vi "JTAG Program.vi"(7 "File format":i32(ring)=1 items=["TI "=1, "Motorola"=2, "Intel"=3], 8 "error in (no error)":errorcluster, 9 "MD5 message-digest":string, 10 "Function":T1(ring), 11 "File Path":path=path "C:/ATS Development/Code/Drivers/JTAG/JTAG Driver/Firmware/Test_Firmware_V1.txt") -> (0 "error out":errorcluster, 1 "MD5 message-digest 2":string, 3 "Status":bool)   [LabVIEW 2010]
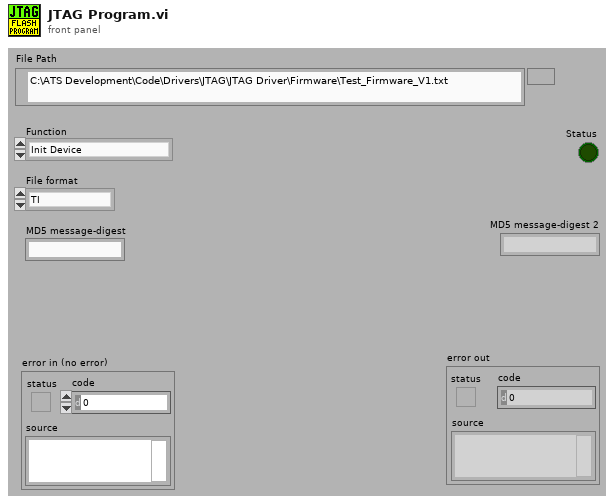
[diagram p1: front panel]
types:
  T1 = enum16{"Init Device", "Auto-Program from File", "Load New Code File", "Close Device", "Blank Check Device", "Erase Device Flash", "Program File to Flash", "Verify Flash vs File", "Read Flash to File", "Checksum of File", "Compare Checksums"}
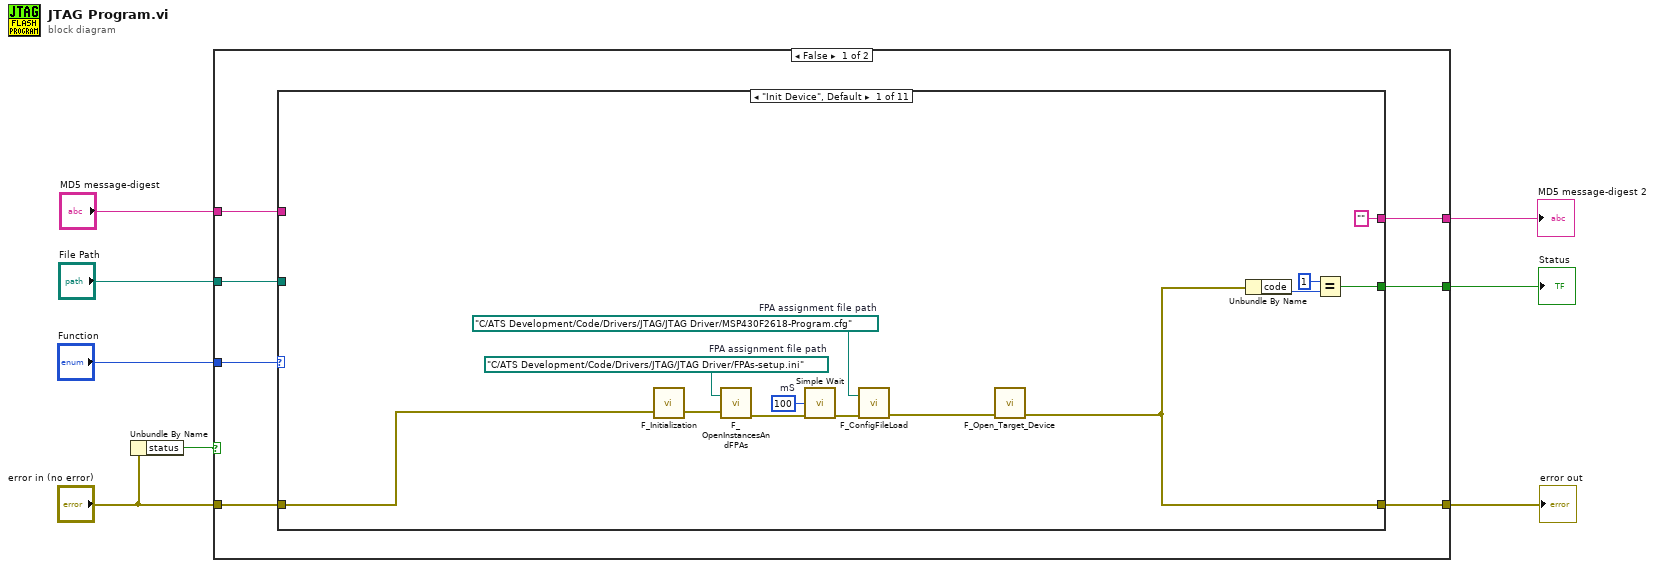
[diagram p0: block diagram]
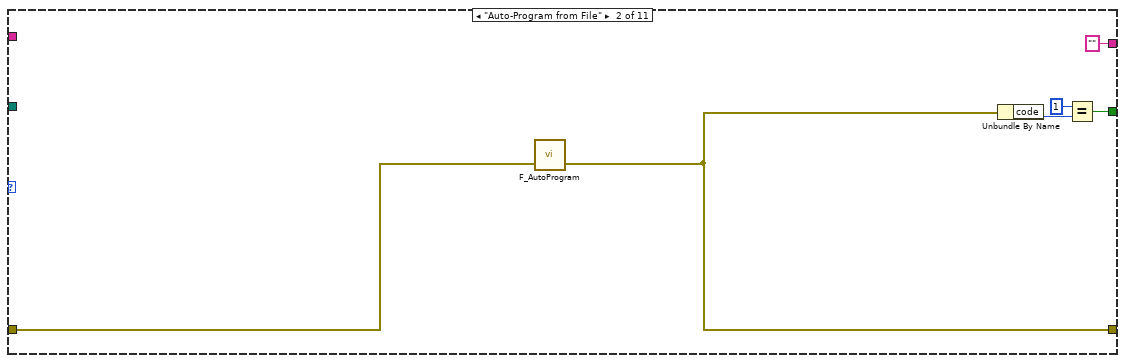
[diagram p2: hidden frame]
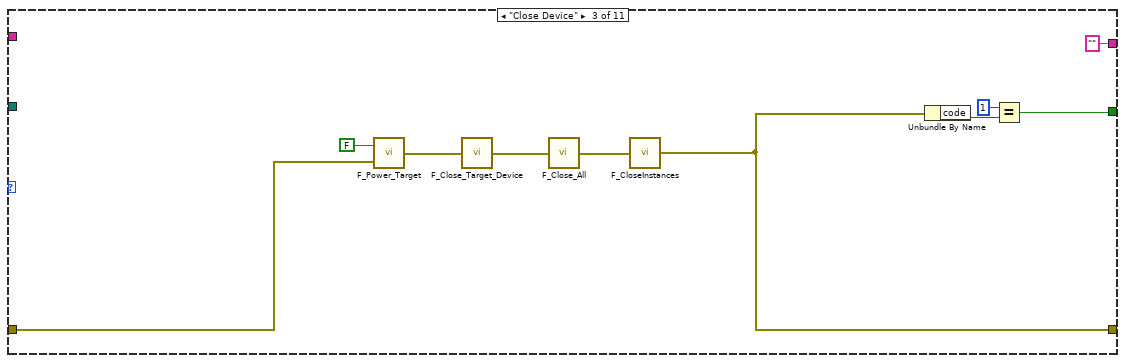
[diagram p3: hidden frame]
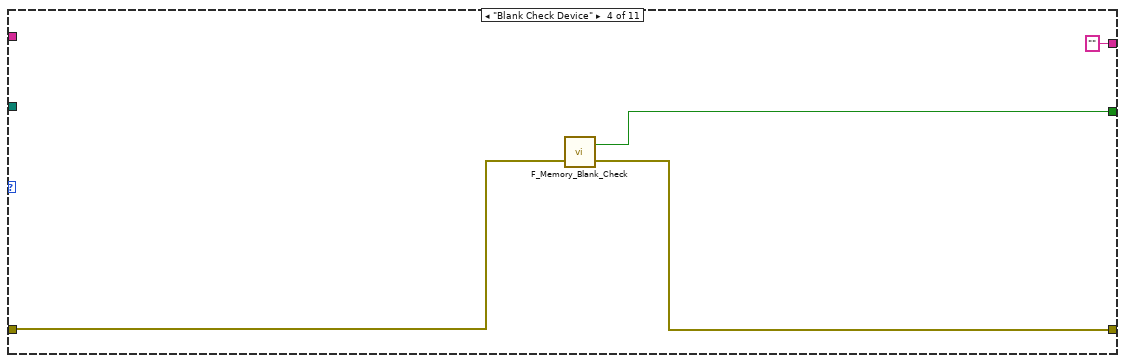
[diagram p4: hidden frame]
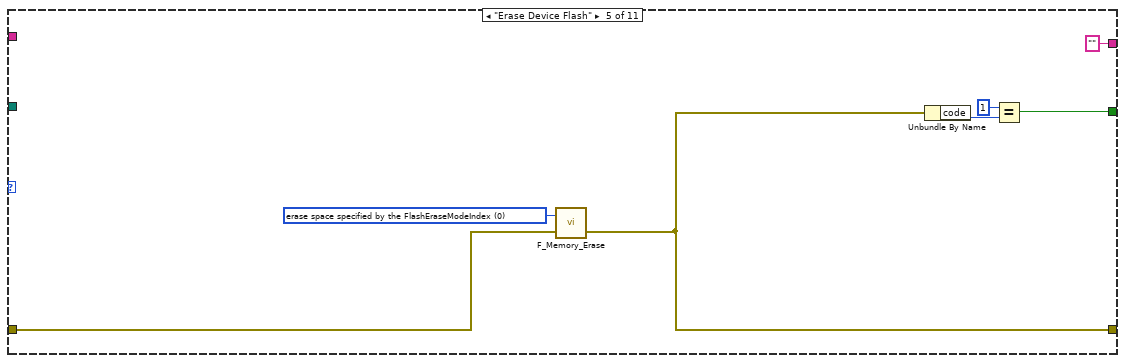
[diagram p5: hidden frame]
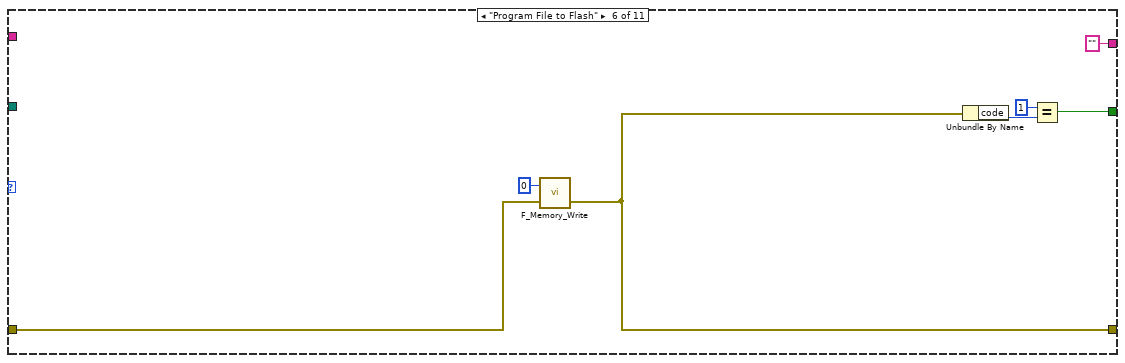
[diagram p6: hidden frame]
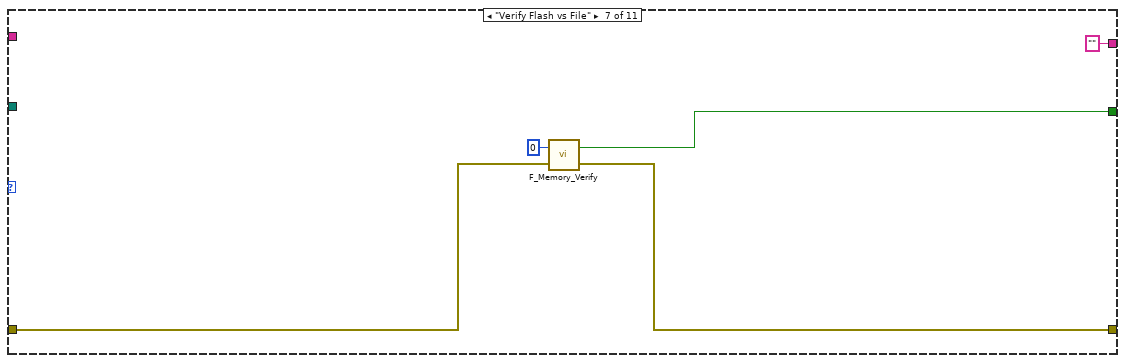
[diagram p7: hidden frame]
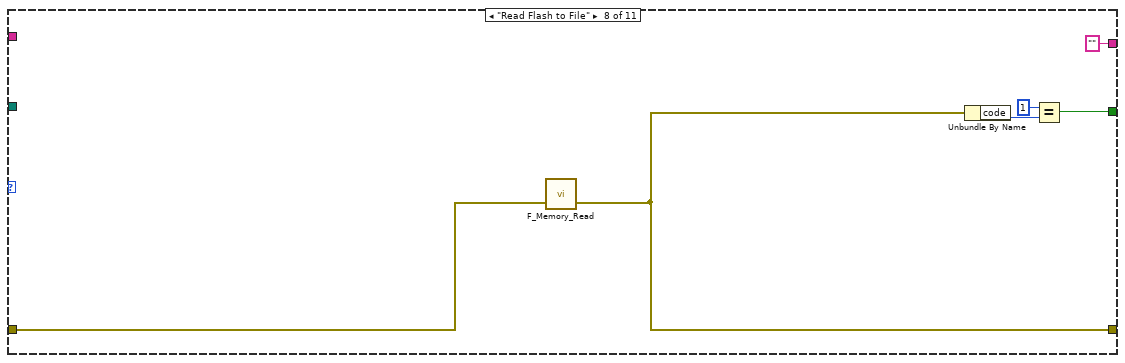
[diagram p8: hidden frame]
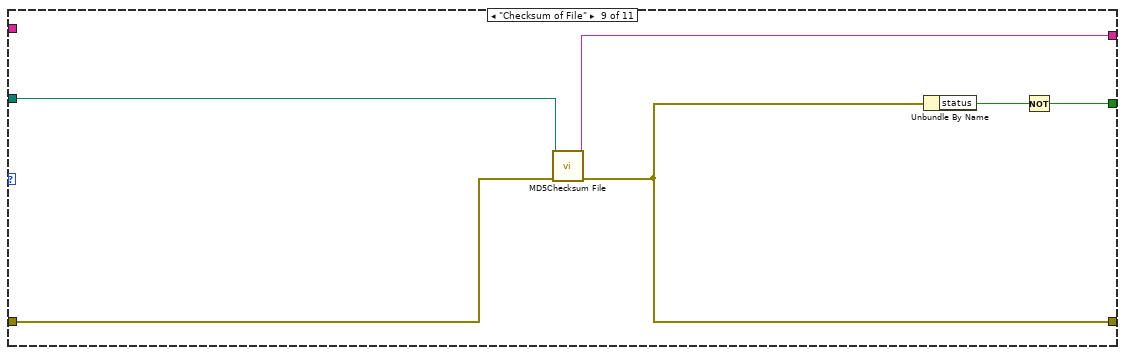
[diagram p9: hidden frame]
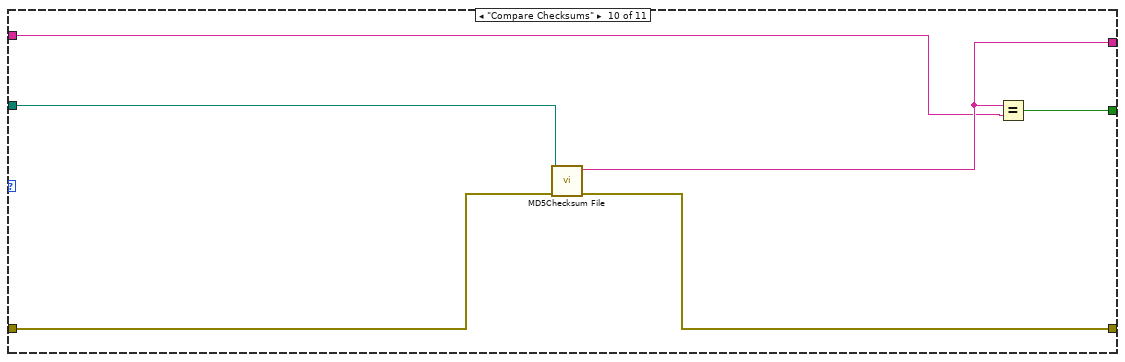
[diagram p10: hidden frame]
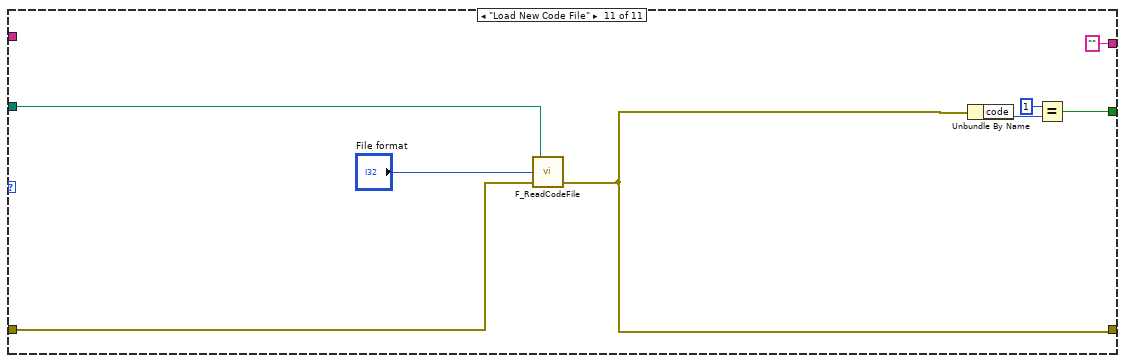
[diagram p11: hidden frame]
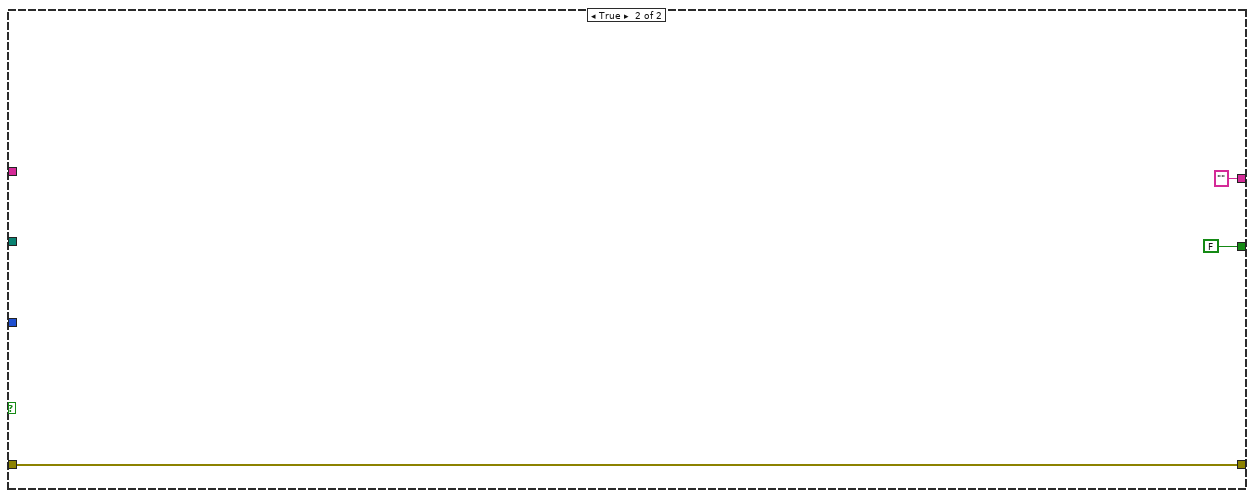
[diagram p12: hidden frame]
diagram:
  n1 = Unbundle By Name("error in (no error)") -> ("status"=w7:bool)
  n2 = case shown="False" w7 {
    tunnel: [w14 w96] -> w8
    tunnel: "error in (no error)" -> [w15 w96]
    tunnel: "MD5 message-digest" -> [w9 _]
    tunnel: "File Path" -> [w10 _]
    tunnel: "Function" -> [w11 _]
    tunnel: [w13 "" ("MD5 message-digest")] -> w2
    tunnel: [w12 FALSE ("Verified")] -> w1
    frame False {
      # "This will be executed if no error exists"
      n3 = case shown="\"Init Device\", Default" w11 {
        tunnel: w15 -> [w22 w33 w36 w48 w55 w62 w67 w73 w79 w81 w92]
        tunnel: [w17 w30 w38 w47 w49 w56 w66 w69 w76 w80 w87] -> w14
        tunnel: ["" ("MD5 message-digest") "" ("MD5 message-digest") "" ("MD5 message-digest") "" ("MD5 message-digest") "" ("MD5 message-digest") "" ("MD5 message-digest") "" ("MD5 message-digest") "" ("MD5 message-digest") w75 w83 "" ("MD5 message-digest")] -> w13
        tunnel: [w16 w29 w41 w46 w50 w57 w64 w68 w78 w84 w88] -> w12
        tunnel: w10 -> [_ _ _ _ _ _ _ _ w74 w85 w93]
        tunnel: w9 -> [_ _ _ _ _ _ _ _ _ w82 _]
        frame "Init Device", Default {
          w27 = path "C:/ATS Development/Code/Drivers/JTAG/JTAG Driver/MSP430F2618-Program.cfg"  # FPA assignment file path
          w25 = u32 100  # mS
          w23 = path "C:/ATS Development/Code/Drivers/JTAG/JTAG Driver/FPAs-setup.ini"  # FPA assignment file path
          n4 = call "F_Initialization.vi"("error in (no error)"=w22) -> ("error out"=w28:errorcluster)
          n5 = call "F_OpenInstancesAndFPAs.vi"("error in (no error)"=w28, "FPA assignment file path"=w23) -> ("error out"=w24:errorcluster)  [unwired: 1 out]
          n6 = call "Simple Wait.vi"("mS"=w25, "error in"=w24) -> ("error out"=w26:errorcluster)  [unwired: 12 in, 1 out]
          n7 = call "F_ConfigFileLoad.vi"("error in (no error)"=w26, "Config file path"=w27) -> ("error out"=w20:errorcluster)  [unwired: 1 in]
          n8 = call "F_Open_Target_Device.vi"("error in (no error)"=w20) -> ("error out"=w17:errorcluster)
          n9 = Unbundle By Name(w17) -> ("code"=w19:i32)
          n10 = Equal?(x=1, y=w19) -> (x = y?=w16:bool)
        }
        frame "Auto-Program from File" {
          n11 = call "F_AutoProgram.vi"("error in (no error)"=w33) -> ("error out"=w30:errorcluster)  [unwired: 2 in]
          n12 = Unbundle By Name(w30) -> ("code"=w32:i32)
          n13 = Equal?(x=1, y=w32) -> (x = y?=w29:bool)
        }
        frame "Close Device" {
          n14 = call "F_Power_Target.vi"("error in (no error)"=w36, "Power Target Device"=FALSE) -> ("error out"=w37:errorcluster)  [unwired: 1 in]
          n15 = call "F_Close_Target_Device.vi"("error in (no error)"=w37) -> ("error out"=w39:errorcluster)
          n16 = call "F_Close_All.vi"("error in (no error)"=w39) -> ("error out"=w40:errorcluster)
          n17 = call "F_CloseInstances.vi"("error in (no error)"=w40) -> ("error out"=w38:errorcluster)
          n18 = Unbundle By Name(w38) -> ("code"=w43:i32)
          n19 = Equal?(x=1, y=w43) -> (x = y?=w41:bool)
        }
        frame "Blank Check Device" {
          n20 = call "F_Memory_Blank_Check.vi"("error in (no error)"=w48) -> ("error out"=w47:errorcluster, "Blank Check"=w46:bool)  [unwired: 1 in]
        }
        frame "Erase Device Flash" {
          w53 = 0 items=["erase space specified by the FlashEraseModeIndex", "erase all Flash memory"] ("Mode of Operation")
          n21 = call "F_Memory_Erase.vi"("error in (no error)"=w55, "Mode of Operation"=w53) -> ("error out"=w49:errorcluster)  [unwired: 1 in]
          n22 = Unbundle By Name(w49) -> ("code"=w52:i32)
          n23 = Equal?(x=1, y=w52) -> (x = y?=w50:bool)
        }
        frame "Program File to Flash" {
          n24 = call "F_Memory_Write.vi"("error in (no error)"=w62, "Mode of Operation"=0) -> ("error out"=w56:errorcluster)  [unwired: 1 in]
          n25 = Unbundle By Name(w56) -> ("code"=w59:i32)
          n26 = Equal?(x=1, y=w59) -> (x = y?=w57:bool)
        }
        frame "Verify Flash vs File" {
          n27 = call "F_Memory_Verify.vi"("error in (no error)"=w67, "Mode of Operation"=0) -> ("error out"=w66:errorcluster, "Verified"=w64:bool)
        }
        frame "Read Flash to File" {
          n28 = call "F_Memory_Read.vi"("error in (no error)"=w73) -> ("error out"=w69:errorcluster)  [unwired: 1 in, 1 out]
          n29 = Unbundle By Name(w69) -> ("code"=w71:i32)
          n30 = Equal?(x=1, y=w71) -> (x = y?=w68:bool)
        }
        frame "Checksum of File" {
          n31 = call <vilib>:"MD5Checksum File.vi"("error in (no error)"=w79, "Path"=w74) -> ("error out"=w76:errorcluster, "MD5 message-digest"=w75:string)  [unwired: 8 in]
          n32 = Unbundle By Name(w76) -> ("status"=w77:bool)
          n33 = Not(x=w77) -> (.not. x?=w78:bool)
        }
        frame "Compare Checksums" {
          n34 = call <vilib>:"MD5Checksum File.vi"("error in (no error)"=w81, "Path"=w85) -> ("error out"=w80:errorcluster, "MD5 message-digest"=w83:string)  [unwired: 8 in]
          n35 = Equal?(x=w83, y=w82) -> (x = y?=w84:bool)
        }
        frame "Load New Code File" {
          n36 = call "F_ReadCodeFile.vi"("error in (no error)"=w92, "File format"="File format", "Code file path"=w93) -> ("error out"=w87:errorcluster)  [unwired: 2 in]
          n37 = Unbundle By Name(w87) -> ("code"=w90:i32)
          n38 = Equal?(x=1, y=w90) -> (x = y?=w88:bool)
        }
      }
    }
    frame True {
      # "Error exists, skip all functions"
    }
  }
  "error out" <- w8
  "Status" <- w1
  "MD5 message-digest 2" <- w2
